vi "HipExo.vi"() -> ()   [LabVIEW 2021]
uses:
  <vilib>/myRIO/Instrument Drivers/Onboard IO/I2C/typedefs/I2C User Configuration.ctl
  <vilib>/myRIO/Instrument Drivers/Onboard IO/I2C/typedefs/I2C Transfer Rate.ctl
  state_typedef.ctl
  <vilib>/Platform/TimedLoop/XDataNode/timing_clust.ctl
  <vilib>/Platform/TimedLoop/XDataNode/nitl_modes.ctl
  <vilib>/Platform/TimedLoop/XDataNode/wakeup.ctl
  <vilib>/myRIO/Instrument Drivers/Onboard IO/PWM/typedefs/PWM Reference.ctl
  <vilib>/myRIO/Common/Instrument Driver Framework/Utilities/typedefs/myRIO Generic Hardware Reference.ctl
  <vilib>/myRIO/Common/Instrument Driver Framework/Utilities/typedefs/Hardware Version Enum.ctl
  <vilib>/myRIO/Common/Instrument Driver Framework/Utilities/typedefs/myRIO v1.0 Reference.ctl
  <vilib>/myRIO/Common/Instrument Driver Framework/Utilities/typedefs/Generic FPGA Reference.ctl
  <vilib>/myRIO/Common/Instrument Driver Framework/myRIO v1.0/PWM/typedefs/PWM Channels Enum.ctl
  <vilib>/myRIO/Instrument Drivers/Onboard IO/PWM/typedefs/PWM Configuration.ctl
  <vilib>/userDefined/High Color/nirio_resource_hc.ctl
  <vilib>/myRIO/Common/Instrument Driver Framework/Utilities/vis/Is FPGA Ref Available.vi
  <vilib>/myRIO/Common/Instrument Driver Framework/myRIO v1.0/PWM/vis/myRIO v1.1 Open PWM.vi
  <vilib>/myRIO/Instrument Drivers/Onboard IO/PWM/vis/Set Duty Cycle and Frequency.vi
  <vilib>/myRIO/Common/Instrument Driver Framework/myRIO v1.0/DIO/vis/myRIO v1.1 Open DIO.vi
  <vilib>/myRIO/Common/Instrument Driver Framework/myRIO v1.0/I2C/vis/myRIO v1.1 Open I2C.vi
  <vilib>/myRIO/Common/Instrument Driver Framework/Utilities/vis/Validate Channels.vi
  <vilib>/myRIO/Common/Instrument Driver Framework/myRIO v1.0/PWM/vis/myRIO v1.0 Reserve PWM.vi
  <vilib>/myRIO/Common/Instrument Driver Framework/myRIO v1.0/UART/vis/myRIO v1.0 Close UART.vi
  <vilib>/myRIO/Common/Instrument Driver Framework/myRIO v1.0/DIO/vis/myRIO v1.0 Reserve DIO.vi
  <vilib>/myRIO/Common/Instrument Driver Framework/myRIO v1.0/I2C/vis/myRIO v1.0 Reserve I2C.vi
  <vilib>/myRIO/Common/Instrument Driver Framework/myRIO v1.0/PWM/vis/myRIO v1.0 Build MUX Configuration PWM.vi
  <vilib>/myRIO/Common/Instrument Driver Framework/myRIO v1.0/Resource Manager/vis/myRIO v1.0 Reserve Channel List.vi
  <vilib>/myRIO/Common/Instrument Driver Framework/myRIO v1.0/DIO/vis/myRIO v1.0 Build MUX Configuration DIO.vi
  <vilib>/myRIO/Common/Instrument Driver Framework/myRIO v1.0/I2C/vis/myRIO v1.0 Build MUX Configuration I2C.vi
  <vilib>/myRIO/Common/Instrument Driver Framework/myRIO v1.0/Resource Manager/vis/myRIO v1.0 Create Configuration List.vi
  <vilib>/myRIO/Common/Instrument Driver Framework/myRIO v1.0/Resource Manager/vis/myRIO v1.0 Reserve Channel.vi
  <vilib>/myRIO/Common/Instrument Driver Framework/myRIO v1.0/Resource Manager/vis/myRIO v1.0 Unreserve Channel.vi
  <vilib>/myRIO/Common/Instrument Driver Framework/myRIO v1.0/Resource Manager/vis/myRIO v1.0 Build Mutex Name.vi
  <vilib>/Utility/VariantDataType/GetNumericInfo.vi
  <vilib>/Utility/error.llb/Error Cluster From Error Code.vi
  <vilib>/myRIO/Common/Instrument Driver Framework/myRIO v1.0/myRIO v1.1 Open.vi
  <vilib>/myRIO/Common/Instrument Driver Framework/Utilities/vis/IO Manager.vi
  <vilib>/myRIO/Common/Instrument Driver Framework/Utilities/vis/Configuration Manager.vi
  <vilib>/myRIO/Common/Instrument Driver Framework/myRIO v1.0/Resource Manager/vis/myRIO v1.0 Configure IO.vi
  <vilib>/myRIO/Common/Instrument Driver Framework/myRIO v1.0/myRIO v1.0 Close.vi
  <vilib>/myRIO/Common/Instrument Driver Framework/myRIO v1.0/I2C/vis/myRIO v1.0 Configure I2C.vi
  <vilib>/myRIO/Common/Instrument Driver Framework/myRIO v1.0/I2C/vis/myRIO v1.0 Write I2C.vi
  <vilib>/myRIO/Common/Instrument Driver Framework/myRIO v1.0/DIO/vis/myRIO v1.0 Write DIO.vi
  <vilib>/myRIO/Common/Instrument Driver Framework/myRIO v1.0/PWM/vis/myRIO v1.0 Write PWM.vi
  <vilib>/myRIO/Common/Instrument Driver Framework/Utilities/vis/FPGA Ref Manager.vi
  <vilib>/myRIO/Common/Instrument Driver Framework/myRIO v1.0/myRIO v1.0 Reset FPGA.vi
  <vilib>/myRIO/Common/Instrument Driver Framework/myRIO v1.0/IRQ/vis/myRIO v1.0 IRQ Info FGV.vi
  <vilib>/myRIO/Common/Instrument Driver Framework/myRIO v1.0/IRQ/vis/myRIO v1.0 Timer IRQ Info FGV.vi
  <vilib>/myRIO/Common/Instrument Driver Framework/myRIO v1.0/IRQ/vis/myRIO v1.0 ISR Agent.vi
  <vilib>/myRIO/Instrument Drivers/Utilities/vis/Reset Index.vi
  <vilib>/myRIO/Common/Instrument Driver Framework/myRIO v1.0/Resource Manager/vis/myRIO v1.0 Block Write Resource Manager.vi
  <vilib>/Platform/TimedLoop/XDataNode/XDataNode.xnode
  <vilib>/myRIO/Express VI/Onboard IO/PWM/PWM Express VI.xnode
  <vilib>/myRIO/Instrument Drivers/Onboard IO/PWM/vis/myRIO PWM Open.xnode
  <vilib>/myRIO/Instrument Drivers/Onboard IO/I2C/I2C.lvlib
  <vilib>/myRIO/Instrument Drivers/Utilities/Utilities.lvlib
  <vilib>/myRIO/Instrument Drivers/Onboard IO/DIO/DIO.lvlib
  <vilib>/Platform/TimedLoop/XDataNode/XDNodeRunTimeDep.lvlib
  <vilib>/myRIO/Instrument Drivers/Onboard IO/PWM/PWM.lvlib
panel:
  out "Numeric":dbl
  in  "error in (no error)":errorcluster
  in  "reset integrator 2":bool
  out "Z displacement 2":dbl format="%#_5g"
  out "Y displacement 2":dbl format="%#_5g"
  out "X displacement 2":dbl format="%#_5g"
  out "Angular displacement [LSB] 2":cluster{dbl, dbl, dbl, dbl}(graph)
  out "Angular rate [LSB/sec] 2":T1(graph)
  out "Z rate 2":dbl format="%.2f"
  out "Y rate 2":dbl format="%.2f"
  out "X rate 2":dbl format="%.2f"
  in  "[ESC]":bool
  out "X":i16
  out "Y":i16
  out "Z":i16
  out "Accelerometer Readings":cluster{i16, i16, i16}(graph)
  out "INT_SOURCE":bool[](array[boolean])
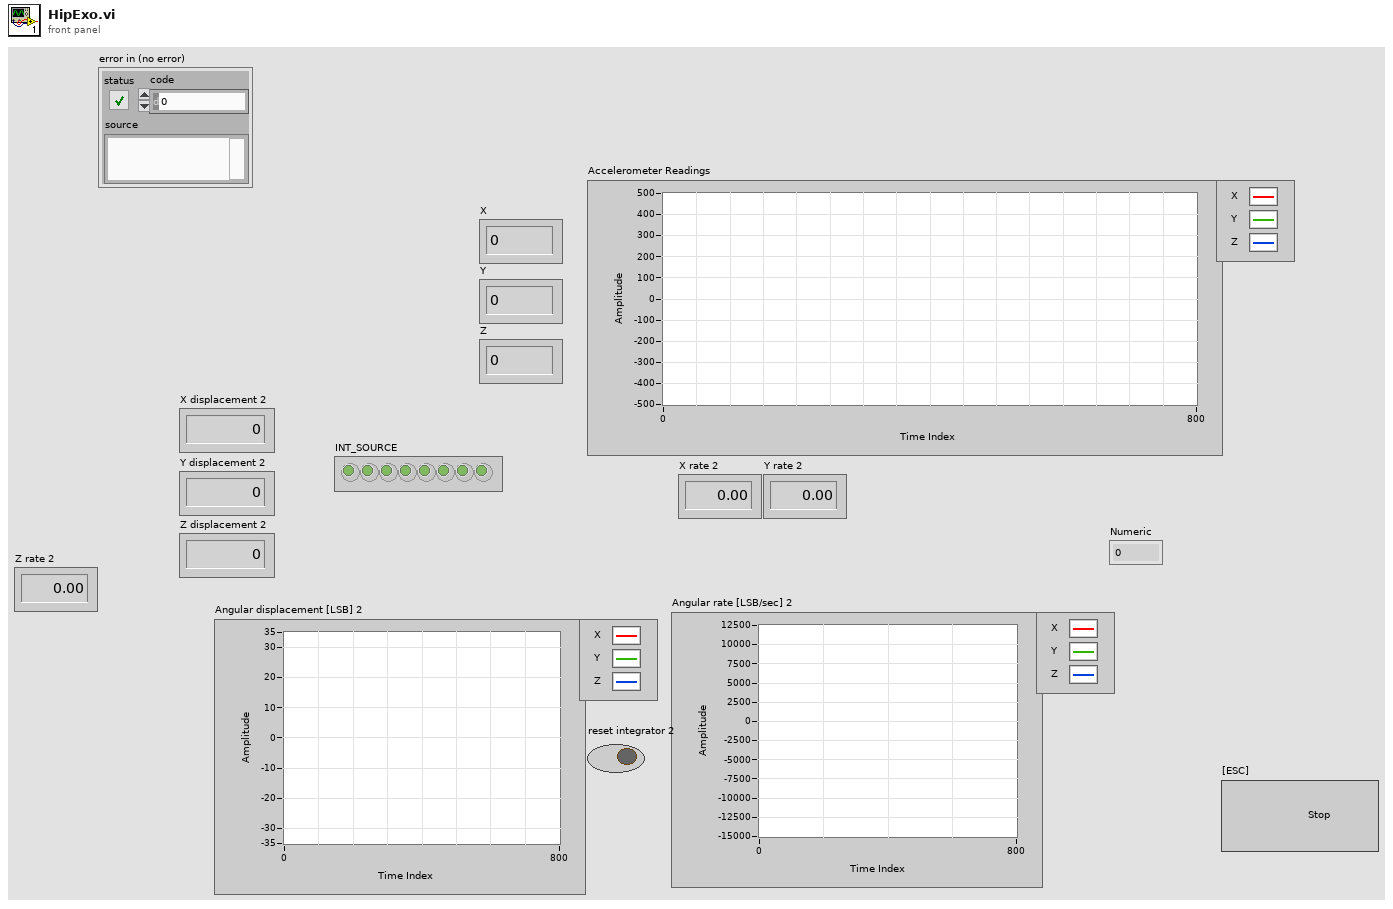
[diagram p1: front panel]
types:
  T1 = cluster{"Numeric 3":dbl, "Numeric 2":dbl, "Numeric":dbl}
  T2 = typedef "state_typedef.ctl" = enum16{"Stair Down", "Stair Up", "Level Walking"}
  T3 = typedef "I2C.lvlib/I2C User Configuration.ctl" = cluster{"I2C Transfer Rate":T4}
  T4 = typedef "I2C.lvlib/I2C Transfer Rate.ctl" = enum16{"Standard mode (100 kbps)", "Fast mode (400 kbps)"}
  T5 = typedef "I2C.lvlib/I2C Reference.ctl" = cluster{"myRIO Reference":T6, "I2C Channels Enum":T10, "I2C Configuration":T11}
  T6 = typedef "myRIO Generic Hardware Reference.ctl" = cluster{"myRIO Model":T7, "myRIO Hardware Reference":T8}
  T7 = typedef "Hardware Version Enum.ctl" = enum16{"Unknown", "myRIO-1900", "myRIO-1950", "roboRIO", "NI ELVIS RIO CM", "ELVIS III"}
  T8 = typedef "myRIO v1.0 Reference.ctl" = cluster{"Generic FPGA Reference":T9, "Allow multiple opens":bool}
  T9 = typedef "Generic FPGA Reference.ctl" = refnum<k20>
  T10 = typedef "I2C Channels Enum.ctl" = enum16{"Not Connected", "A/I2C", "B/I2C", "I2C/I2C"}
  T11 = typedef "I2C.lvlib/I2C Configuration.ctl" = cluster{"I2C Transfer Rate":T4}
  T12 = typedef "DIO.lvlib/DIO Reference.ctl" = cluster{"myRIO Reference":T6, "DIO Channels List":T13}
  T13 = typedef "DIO Channels List.ctl" = T14[]
  T14 = typedef "DIO Channels Enum.ctl" = enum16{"Not Connected", "C/DIO0", "C/DIO1", "C/DIO2", "C/DIO3", "C/DIO4", "C/DIO5", "C/DIO6", "C/DIO7", "A/DIO0", "A/DIO1", "A/DIO2", "A/DIO3", "A/DIO4", "A/DIO5", "A/DIO6", "A/DIO7", "A/DIO8", "A/DIO9", "A/DIO10", "A/DIO11", "A/DIO12", "A/DIO13", "A/DIO14", "A/DIO15", "A/DIO16", "A/DIO17", "A/DIO18", "A/DIO19", "B/DIO0", "B/DIO1", "B/DIO2", "B/DIO3", "B/DIO4", "B/DIO5", "B/DIO6", "B/DIO7", "B/DIO8", "B/DIO9", "B/DIO10", "B/DIO11", "B/DIO12", "B/DIO13", "B/DIO14", "B/DIO15", "B/DIO16", "B/DIO17", "B/DIO18", "B/DIO19", "LED0", "LED1", "LED2", "LED3", "Button0", "DIO/DIO0", "DIO/DIO1", "DIO/DIO2", "DIO/DIO3", "DIO/DIO4", "DIO/DIO5", "DIO/DIO6", "DIO/DIO7", "DIO/DIO8", "DIO/DIO9", "SPI/CS0", "SPI/CS1", "SPI/CS2", "SPI/CS3", "LED RADIO (Green)", "LED RADIO (Red)", "LED COMM (Green)", "LED COMM (Red)", "LED MODE (Green)", "LED MODE (Red)"}
  T15 = typedef "XDNodeRunTimeDep.lvlib/timing_clust.ctl" = cluster{"Expected End [f-1]":u64, "Actual End [f-1]":u64, "Finished Late? [f-1]":bool, "Expected End [i-1]":u64, "Actual End [i-1]":u64, "Finished Late? [i-1]":bool, "Expected Start [i]":u64, "Actual Start [i]":u64, "Expected Start [f]":u64, "Actual Start [f]":u64, "Source Name":string, "Structure Name":string, "Period":i64, "Deadline":i64, "Offset":i64, "Start":i64, "Priority":i32, "Timeout":i32, "Mode":T16, "Wakeup Reason":T17, "Error":errorcluster, "Source Type":string, "Secondary Source Type":string, "Global End Time":u64, "Global Start Time":u64, "Frame Duration":u64, "Iteration Duration":u64, "Assigned CPU":i32, "I/O Scan Engine Mode":u32}
  T16 = typedef "XDNodeRunTimeDep.lvlib/nitl_modes.ctl" = enum32{"No Change", "Process missed periods, maintain original phase", "Discard missed periods, maintain original phase", "Process missed periods, ignore original phase", "Discard missed periods, ignore original phase"}
  T17 = typedef "XDNodeRunTimeDep.lvlib/wakeup.ctl" = enum32{"Normal", "Aborted", "Asynchronous wakeup", "Timing source error", "Timed loop error", "Timeout"}
  T18 = typedef "PWM.lvlib/PWM Reference.ctl" = cluster{"myRIO Reference":T6, "PWM Channels Enum":T19, "PWM Configuration":T20}
  T19 = typedef "PWM Channels Enum.ctl" = enum16{"Not Connected", "C/PWM0", "C/PWM1", "A/PWM0", "A/PWM1", "A/PWM2", "A/PWM3", "A/PWM4", "A/PWM5", "A/PWM6", "A/PWM7", "A/PWM8", "A/PWM9", "A/PWM10", "A/PWM11", "A/PWM12", "A/PWM13", "A/PWM14", "A/PWM15", "A/PWM16", "A/PWM17", "A/PWM18", "A/PWM19", "B/PWM0", "B/PWM1", "B/PWM2", "B/PWM3", "B/PWM4", "B/PWM5", "B/PWM6", "B/PWM7", "B/PWM8", "B/PWM9", "B/PWM10", "B/PWM11", "B/PWM12", "B/PWM13", "B/PWM14", "B/PWM15", "B/PWM16", "B/PWM17", "B/PWM18", "B/PWM19", "PWM/PWM0", "PWM/PWM1", "PWM/PWM2", "PWM/PWM3", "PWM/PWM4", "PWM/PWM5", "PWM/PWM6", "PWM/PWM7", "PWM/PWM8", "PWM/PWM9"}
  T20 = typedef "PWM.lvlib/PWM Configuration.ctl" = cluster{"Frequency":dbl, "Duty Cycle":dbl}
  T21 = typedef "nirio_resource_hc.ctl" = tag
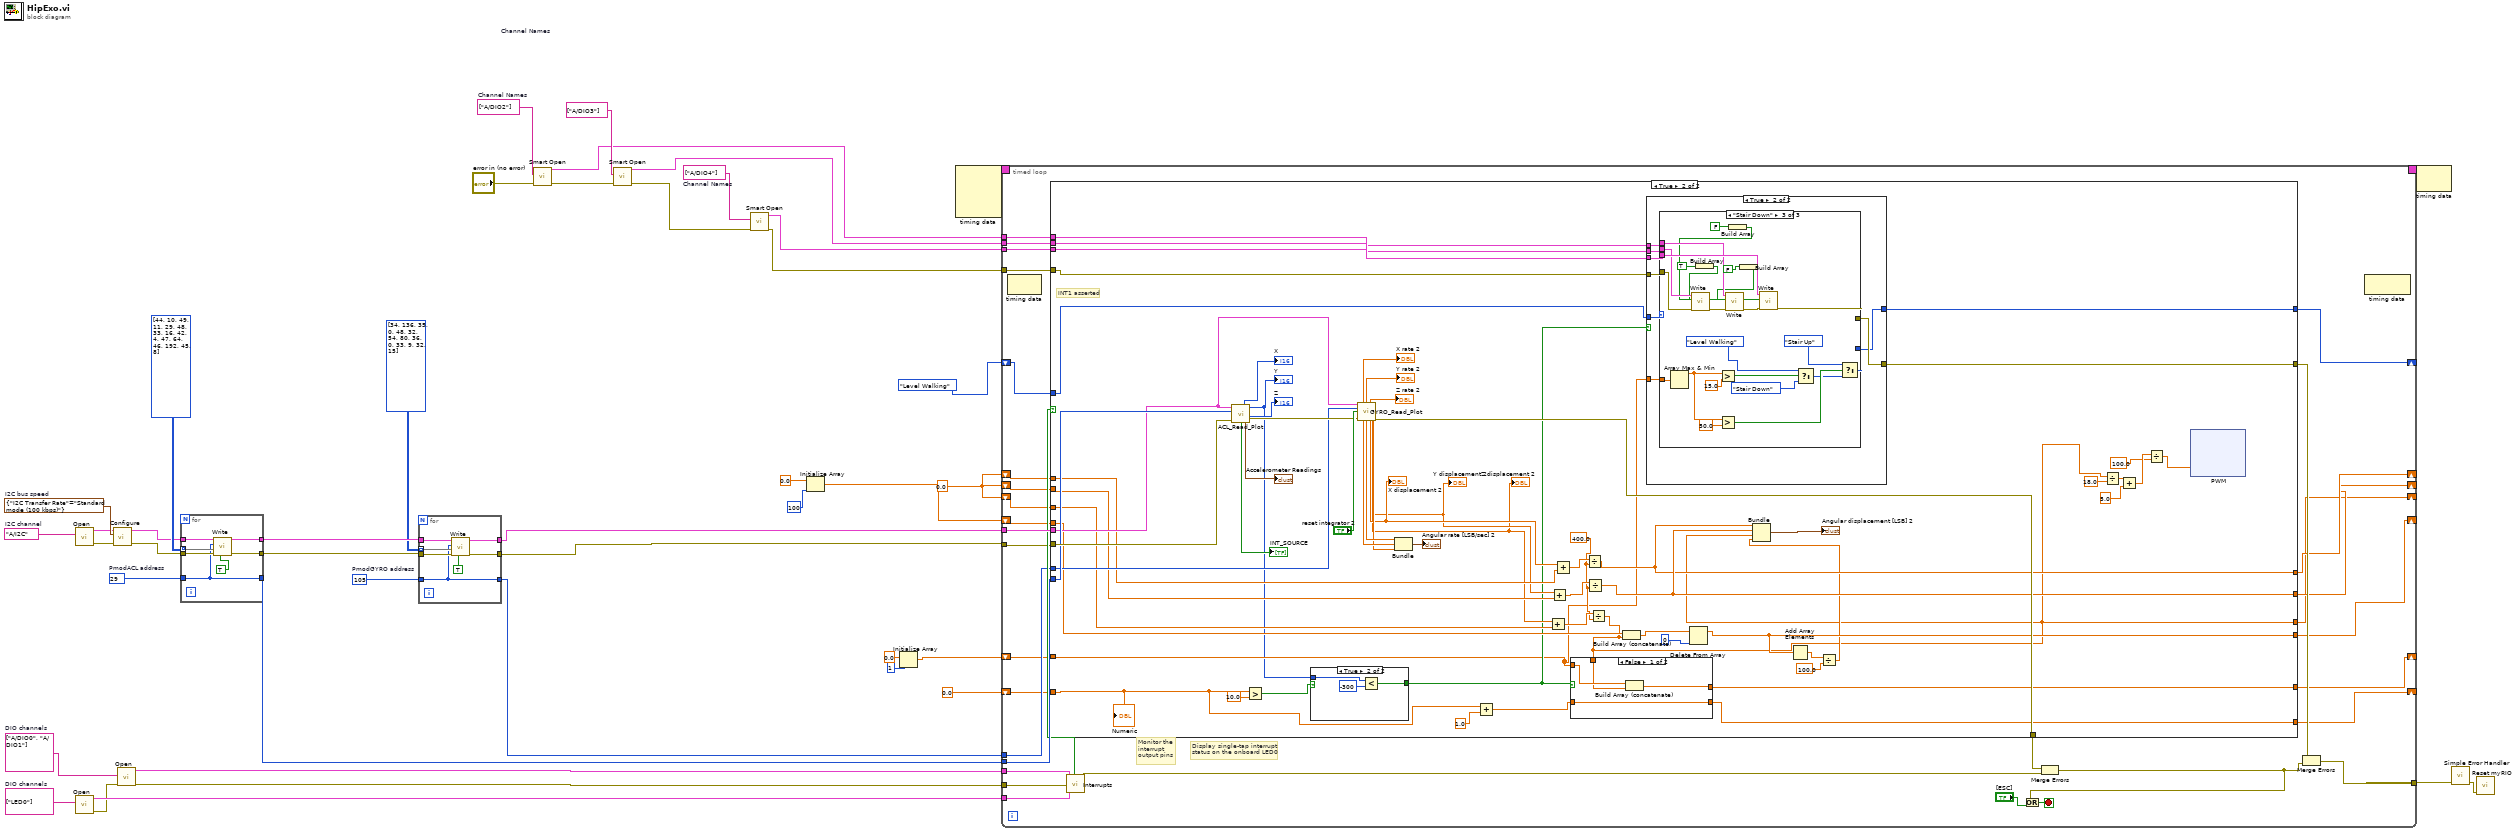
[diagram p0: block diagram]
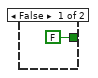
[diagram p3: hidden frame]
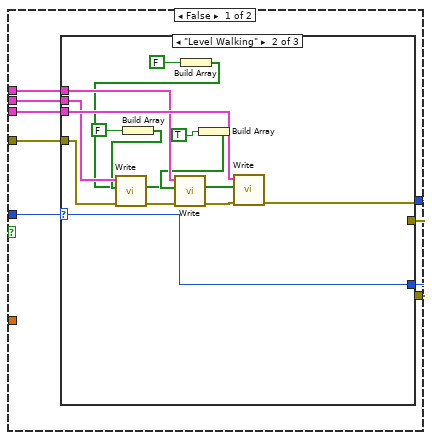
[diagram p4: hidden frame]
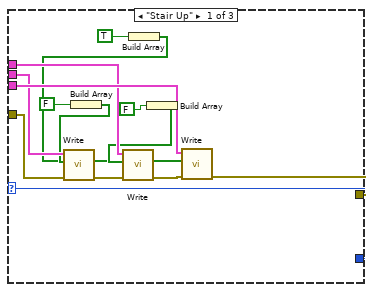
[diagram p5: hidden frame]
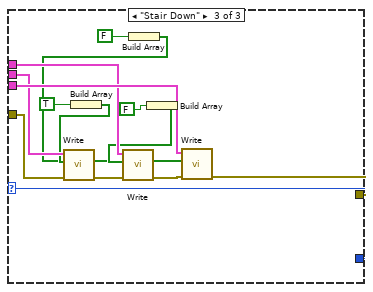
[diagram p6: hidden frame]
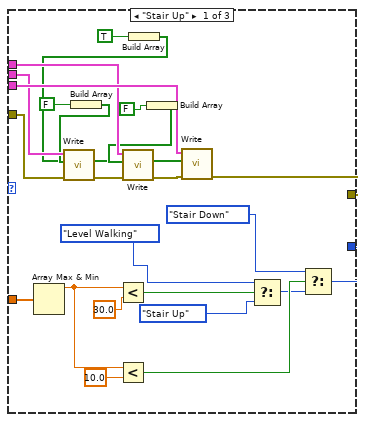
[diagram p7: hidden frame]
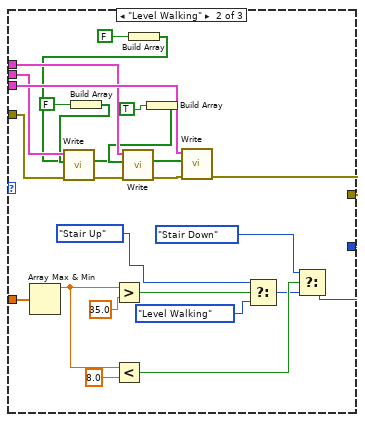
[diagram p8: hidden frame]
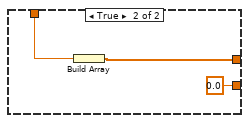
[diagram p9: hidden frame]
diagram:
  w9 = 0.0
  w16 = tag[] ["A/DIO3"]  # Channel Names
  w17 = tag[] ["A/DIO4"]  # Channel Names
  w19 = tag[] ["A/DIO2"]  # Channel Names
  w23 = u8 105  # PmodGYRO address
  w29 = tag[] ["LED0"]  # DIO channels
  w30 = tag[] ["A/DIO0", "A/DIO1"]  # DIO channels
  w40 = T3 {"I2C Transfer Rate"=enum."Standard mode (100 kbps)"}  # I2C bus speed
  w41 = tag "A/I2C"  # I2C channel
  w33 = u8 29  # PmodACL address
  n1 = call <vilib>:"Open.vi"("Channel Name"=w41) -> ("error out"=w38:errorcluster, "I2C Ref Out"=w39:T5)  [unwired: 9 in]
  n2 = call <vilib>:"Open.vi"("Channel Names"=w29) -> ("error out"=w27:errorcluster, "DIO Ref Out"=w28:T12)  [unwired: 9 in]
  n3 = call <vilib>:"Configure.vi"("error in (no error)"=w38, "I2C User Configuration"=w40, "I2C Ref In"=w39) -> ("error out"=w34:errorcluster, "I2C Ref Out"=w35:T5)  [unwired: 7 in]
  n4 = call <vilib>:"Open.vi"("error in (no error)"=w27, "Channel Names"=w30) -> ("error out"=w32:errorcluster, "DIO Ref Out"=w31:T12)  [unwired: 8 in]
  n5 = for {
    tunnel: [w52] -> w25
    tunnel: [w51] -> w26
    tunnel: [w47] -> w37
    tunnel: u8[][] [[44, 10], [49, 11], [29, 48], [33, 16], [42, 4], [47, 64], [46, 192], [45, 8]] ("Bytes to Write") -> [w50] mode=indexing
    tunnel: w35 -> [w49]
    tunnel: w34 -> [w48]
    tunnel: w33 -> [w47]
    n6 = call <vilib>:"Write.vi"("Keep Bus Busy"=TRUE, "error in (no error)"=w48, "Bytes to Write"=w50, "Slave Address (7-bit)"=w47, "I2C Ref In"=w49) -> ("error out"=w52:errorcluster, "I2C Ref Out"=w51:T5)  [unwired: 5 in]
  }
  n7 = for {
    tunnel: [w59] -> w21
    tunnel: [w58] -> w20
    tunnel: [w54] -> w22
    tunnel: u8[][] [[34, 136], [35, 0], [48, 32], [54, 80], [36, 0], [33, 9], [32, 15]] ("Bytes to Write") -> [w57] mode=indexing
    tunnel: w26 -> [w56]
    tunnel: w25 -> [w55]
    tunnel: w23 -> [w54]
    n8 = call <vilib>:"Write.vi"("Keep Bus Busy"=TRUE, "error in (no error)"=w55, "Bytes to Write"=w57, "Slave Address (7-bit)"=w54, "I2C Ref In"=w56) -> ("error out"=w59:errorcluster, "I2C Ref Out"=w58:T5)  [unwired: 5 in]
  }
  n9 = call <vilib>:"Smart Open.vi"("error in (no error)"="error in (no error)", "Channel Names"=w19) -> ("error out"=w15:errorcluster, "DIO Ref Out"=w10:T12)  [unwired: 8 in]
  n10 = call <vilib>:"Smart Open.vi"("error in (no error)"=w15, "Channel Names"=w16) -> ("error out"=w14:errorcluster, "DIO Ref Out"=w11:T12)  [unwired: 8 in]
  n11 = call <vilib>:"Smart Open.vi"("error in (no error)"=w14, "Channel Names"=w17) -> ("error out"=w13:errorcluster, "DIO Ref Out"=w12:T12)  [unwired: 8 in]
  n12 = Initialize Array(0.0, 100) -> (w6:dbl[])
  n13 = Initialize Array(0.0 ("element"), 1 ("dimension size")) -> (w2:dbl[])
  n14 = node-c288() -> (w45:T15)  [unwired: 4 in]
  n15 = timed-loop {
    tunnel: [w78] -> w42
    tunnel: w37 -> [w89]
    tunnel: w32 -> [w88]
    tunnel: w31 -> [w87]
    timing: w45 -> [_]
    timing-out: [_] -> w44
    tunnel: w28 -> [w84]
    tunnel: w21 -> [w82]
    tunnel: w22 -> [w81]
    shift-right: [w80] -> _
    shift-left: state_typedef."Level Walking" -> [w72]
    tunnel: w13 -> [w79]
    tunnel: w12 -> [w75]
    tunnel: w11 -> [w74]
    tunnel: w10 -> [w73]
    tunnel: w20 -> [w90]
    shift-right: [w70] -> _
    shift-left: w9 -> [w71]
    shift-right: [w67] -> _
    shift-left: w9 -> [w69]
    shift-right: [w66] -> _
    shift-left: w9 -> [w68]
    shift-right: [w64] -> _
    shift-left: w6 -> [w65]
    shift-right: [w62] -> _
    shift-left: w2 -> [w63]
    shift-right: [w60] -> _
    shift-left: 0.0 -> [w61]
    stop <- w92 stop-if-true
    # "Display single-tap interrupt\nstatus on the onboard LED0"
    # "Monitor the\ninterrupt\noutput pins"
    n16 = node-c288() -> ()  [unwired: 1 in, 1 out]
    n17 = call "Interrupts.vi"("error in (no error)"=w88, "DIO Ref Out"=w84, "DIO Ref Out 2"=w87) -> ("error out"=w83:errorcluster, "INT1"=w85:bool)  [unwired: 7 in]
    n18 = case shown="True" w85 {
      tunnel: w82 -> [w103 w164]
      tunnel: w90 -> [_ w150]
      tunnel: w89 -> [_ w163]
      tunnel: [w103 w149] -> w86
      tunnel: w81 -> [_ w151]
      tunnel: w72 -> [w102 w148]
      tunnel: [w102 w147] -> w80
      tunnel: w79 -> [w101 w146]
      tunnel: [w101 w145] -> w76
      tunnel: w75 -> [_ w144]
      tunnel: w74 -> [_ w143]
      tunnel: w73 -> [_ w142]
      tunnel: w71 -> [w100 w141]
      tunnel: [w100 w131] -> w70
      tunnel: w69 -> [w99 w139]
      tunnel: w68 -> [w98 w138]
      tunnel: [w99 w133] -> w67
      tunnel: [w98 w111] -> w66
      tunnel: w65 -> [w97 w129]
      tunnel: [w97 w126] -> w64
      tunnel: w63 -> [w96 w121]
      tunnel: [w96 w114] -> w62
      tunnel: w61 -> [w95 w108]
      tunnel: [w95 w110] -> w60
      frame False {
        # "INT1 deasserted"
      }
      frame True {
        w130 = 400.0
        # "INT1 asserted"
        n19 = call "ACL_Read_Plot.vi"("error in (no error)"=w164, "PmodACL address"=w163, "I2C Ref Out"=w150) -> ("error out"=w152:errorcluster, "Numeric 3"=→"Z":i16, "Array"=→"INT_SOURCE":bool[], "Numeric"=w104:i16, "Cluster"=→"Accelerometer Readings":cluster{i16, i16, i16}, "Numeric 2"=→"X":i16)  [unwired: 3 in]
        "Y" <- w104
        n20 = Greater?(x=w108, y=10.0) -> (0:w113:bool)
        n21 = case shown="True" w113 {
          tunnel: [FALSE w168] -> w122
          tunnel: w104 -> [_ w167]
          frame False {
          }
          frame True {
            n22 = Less?(x=w167, y=i16 -300) -> (x < y?=w168:bool)
          }
        }
        n23 = call "GYRO_Read_Plot.vi"("I2C Ref Out"=w150, "PmodGYRO address"=w151, "reset integrator"="reset integrator 2", "error in (no error)"=w152) -> ("X rate"=→"X rate 2":dbl, "Y rate"=→"Y rate 2":dbl, "integral x(t)"=w140:dbl, "integral x(t) 3"=w137:dbl, "Numeric"=w157:dbl, "integral x(t) 2"=w136:dbl, "Numeric 2"=w158:dbl, "Numeric 3"=w160:dbl, "Z rate"=→"Z rate 2":dbl, "error out"=w149:errorcluster)  [unwired: 1 in, 1 out]
        "X displacement 2" <- w140
        "Y displacement 2" <- w137
        "Z displacement 2" <- w136
        n24 = Bundle "Bundle"("Numeric 3"=w160, "Numeric 2"=w158, "Numeric"=w157) -> (→"Angular rate [LSB/sec] 2":T1)  [unwired: 1 in]
        n25 = Add(x=w108, y=1.0) -> (x+y=w107:dbl)
        n26 = Add(x=w136, y=w138) -> (x+y=w135:dbl)
        n27 = Add(x=w137, y=w139) -> (x+y=w134:dbl)
        n28 = Add(x=w140, y=w141) -> (x+y=w132:dbl)
        n29 = Divide(x=w132, y=w130) -> (x/y=w131:dbl)
        n30 = Divide(x=w134, y=w130) -> (x/y=w133:dbl)
        n31 = Divide(x=w135, y=w130) -> (x/y=w111:dbl)
        n32 = case shown="False" w122 {
          tunnel: w121 -> [w337 _]
          tunnel: w111 -> [w336 w340]
          tunnel: [w335 w339] -> w114
          tunnel: w107 -> [w334 _]
          tunnel: [w334 0.0] -> w110
          frame False {
            n33 = Build Array (concatenate)(w337, w336) -> (w335:dbl[])
          }
          frame True {
            n34 = Build Array(w340) -> (w339:dbl[])
          }
        }
        n35 = Build Array (concatenate)(w129, w111) -> (w128:dbl[])
        n36 = case shown="True" w122 {
          tunnel: w148 -> [w211 w257]
          tunnel: [w210 w255] -> w147
          tunnel: w146 -> [w209 w258]
          tunnel: [w208 w256] -> w145
          tunnel: w144 -> [w207 w259]
          tunnel: w143 -> [w206 w260]
          tunnel: w142 -> [w205 w261]
          tunnel: w121 -> [_ w254]
          frame False {
            n37 = case shown="\"Level Walking\"" w211 {
              selector: w211 -> [w225 w226 w253]
              tunnel: [w225 w226 w253] -> w210
              tunnel: w209 -> [w221 w236 w249]
              tunnel: [w224 w239 w252] -> w208
              tunnel: w207 -> [w223 w238 w251]
              tunnel: w206 -> [w222 w237 w250]
              tunnel: w205 -> [w218 w233 w246]
              frame "Stair Up" {
                n38 = Build Array(FALSE) -> (w216:bool[])
                n39 = call <vilib>:"Write.vi"("error in (no error)"=w221, "Values"=w216, "DIO Ref In"=w222) -> ("error out"=w220:errorcluster)  [unwired: 6 in, 1 out]
                n40 = Build Array(TRUE) -> (w212:bool[])
                n41 = Build Array(FALSE) -> (w214:bool[])
                n42 = call <vilib>:"Write.vi"("error in (no error)"=w220, "Values"=w214, "DIO Ref In"=w218) -> ("error out"=w219:errorcluster)  [unwired: 6 in, 1 out]
                n43 = call <vilib>:"Write.vi"("error in (no error)"=w219, "Values"=w212, "DIO Ref In"=w223) -> ("error out"=w224:errorcluster)  [unwired: 6 in, 1 out]
              }
              frame "Level Walking" {
                n44 = Build Array(FALSE) -> (w231:bool[])
                n45 = call <vilib>:"Write.vi"("error in (no error)"=w236, "Values"=w231, "DIO Ref In"=w237) -> ("error out"=w235:errorcluster)  [unwired: 6 in, 1 out]
                n46 = Build Array(FALSE) -> (w227:bool[])
                n47 = Build Array(TRUE) -> (w229:bool[])
                n48 = call <vilib>:"Write.vi"("error in (no error)"=w235, "Values"=w229, "DIO Ref In"=w233) -> ("error out"=w234:errorcluster)  [unwired: 6 in, 1 out]
                n49 = call <vilib>:"Write.vi"("error in (no error)"=w234, "Values"=w227, "DIO Ref In"=w238) -> ("error out"=w239:errorcluster)  [unwired: 6 in, 1 out]
              }
              frame "Stair Down" {
                n50 = Build Array(TRUE) -> (w244:bool[])
                n51 = call <vilib>:"Write.vi"("error in (no error)"=w249, "Values"=w244, "DIO Ref In"=w250) -> ("error out"=w248:errorcluster)  [unwired: 6 in, 1 out]
                n52 = Build Array(FALSE) -> (w240:bool[])
                n53 = Build Array(FALSE) -> (w242:bool[])
                n54 = call <vilib>:"Write.vi"("error in (no error)"=w248, "Values"=w242, "DIO Ref In"=w246) -> ("error out"=w247:errorcluster)  [unwired: 6 in, 1 out]
                n55 = call <vilib>:"Write.vi"("error in (no error)"=w247, "Values"=w240, "DIO Ref In"=w251) -> ("error out"=w252:errorcluster)  [unwired: 6 in, 1 out]
              }
            }
          }
          frame True {
            n56 = case shown="\"Stair Down\"" w257 {
              tunnel: [w262 w286 w310] -> w255
              tunnel: w258 -> [w282 w306 w330]
              tunnel: [w285 w309 w333] -> w256
              tunnel: w259 -> [w284 w308 w332]
              tunnel: w260 -> [w283 w307 w331]
              tunnel: w261 -> [w279 w303 w327]
              tunnel: w254 -> [w263 w292 w311]
              frame "Stair Up" {
                n57 = Array Max & Min(array=w263) -> (max value=w268:dbl)  [unwired: 3 out]
                n58 = Build Array(FALSE) -> (w277:bool[])
                n59 = call <vilib>:"Write.vi"("error in (no error)"=w282, "Values"=w277, "DIO Ref In"=w283) -> ("error out"=w281:errorcluster)  [unwired: 6 in, 1 out]
                n60 = Less?(x=w268, y=30.0) -> (x < y?=w271:bool)
                n61 = Less?(x=w268, y=10.0) -> (x < y?=w266:bool)
                n62 = Build Array(TRUE) -> (w273:bool[])
                n63 = Build Array(FALSE) -> (w275:bool[])
                n64 = call <vilib>:"Write.vi"("error in (no error)"=w281, "Values"=w275, "DIO Ref In"=w279) -> ("error out"=w280:errorcluster)  [unwired: 6 in, 1 out]
                n65 = call <vilib>:"Write.vi"("error in (no error)"=w280, "Values"=w273, "DIO Ref In"=w284) -> ("error out"=w285:errorcluster)  [unwired: 6 in, 1 out]
                n66 = Select(t=state_typedef."Level Walking", s=w271, f=state_typedef."Stair Up") -> (s? t:f=w264:T2)
                n67 = Select(t=state_typedef."Stair Down", s=w266, f=w264) -> (s? t:f=w262:T2)
              }
              frame "Level Walking" {
                n68 = Array Max & Min(array=w292) -> (max value=w291:dbl)  [unwired: 3 out]
                n69 = Build Array(FALSE) -> (w301:bool[])
                n70 = call <vilib>:"Write.vi"("error in (no error)"=w306, "Values"=w301, "DIO Ref In"=w307) -> ("error out"=w305:errorcluster)  [unwired: 6 in, 1 out]
                n71 = Greater?(x=w291, y=35.0) -> (0:w295:bool)
                n72 = Less?(x=w291, y=8.0) -> (x < y?=w289:bool)
                n73 = Build Array(FALSE) -> (w297:bool[])
                n74 = Build Array(TRUE) -> (w299:bool[])
                n75 = call <vilib>:"Write.vi"("error in (no error)"=w305, "Values"=w299, "DIO Ref In"=w303) -> ("error out"=w304:errorcluster)  [unwired: 6 in, 1 out]
                n76 = call <vilib>:"Write.vi"("error in (no error)"=w304, "Values"=w297, "DIO Ref In"=w308) -> ("error out"=w309:errorcluster)  [unwired: 6 in, 1 out]
                n77 = Select(t=state_typedef."Stair Up", s=w295, f=state_typedef."Level Walking") -> (s? t:f=w287:T2)
                n78 = Select(t=state_typedef."Stair Down", s=w289, f=w287) -> (s? t:f=w286:T2)
              }
              frame "Stair Down" {
                n79 = Array Max & Min(array=w311) -> (max value=w316:dbl)  [unwired: 3 out]
                n80 = Build Array(TRUE) -> (w325:bool[])
                n81 = call <vilib>:"Write.vi"("error in (no error)"=w330, "Values"=w325, "DIO Ref In"=w331) -> ("error out"=w329:errorcluster)  [unwired: 6 in, 1 out]
                n82 = Greater?(x=w316, y=15.0) -> (0:w319:bool)
                n83 = Greater?(x=w316, y=50.0) -> (0:w314:bool)
                n84 = Build Array(FALSE) -> (w321:bool[])
                n85 = Build Array(FALSE) -> (w323:bool[])
                n86 = call <vilib>:"Write.vi"("error in (no error)"=w329, "Values"=w323, "DIO Ref In"=w327) -> ("error out"=w328:errorcluster)  [unwired: 6 in, 1 out]
                n87 = call <vilib>:"Write.vi"("error in (no error)"=w328, "Values"=w321, "DIO Ref In"=w332) -> ("error out"=w333:errorcluster)  [unwired: 6 in, 1 out]
                n88 = Select(t=state_typedef."Level Walking", s=w319, f=state_typedef."Stair Down") -> (s? t:f=w312:T2)
                n89 = Select(t=state_typedef."Stair Up", s=w314, f=w312) -> (s? t:f=w310:T2)
              }
            }
          }
        }
        n90 = Delete From Array(array=w128, index=0) -> (array with subset deleted=w126:dbl[])  [unwired: 1 in, 1 out]
        n91 = Add Array Elements(numeric array=w126) -> (sum=w125:dbl)
        n92 = Divide(x=w125, y=100.0) -> (x/y=w123:dbl)
        n93 = Bundle "Bundle"(w131, w133, w111, w123) -> (→"Angular displacement [LSB] 2":cluster{dbl, dbl, dbl, dbl})  [unwired: 1 in]
        n94 = Divide(x=w111, y=18.0) -> (x/y=w118:dbl)
        n95 = Add(x=w118, y=5.0) -> (x+y=w120:dbl)
        n96 = Divide(x=w120, y=100.0) -> (x/y=w119:dbl)
        n97 = xnode "PWM"("Duty Cycle"=w119) -> ()  [unwired: 1 in, 1 out]
        "Numeric" <- w108
      }
    }
    n98 = Merge Errors "Merge Errors"(w86, w83) -> (w77:errorcluster)
    n99 = Or(x=w77, y="[ESC]") -> (x .or. y?=w92:bool)
    n100 = Merge Errors "Merge Errors"(w76, w77) -> (w78:errorcluster)
    n101 = node-c288() -> ()  [unwired: 1 in, 1 out]
  }
  n102 = node-c288(w44) -> ()  [unwired: 1 out]
  n103 = call <vilib>:"Simple Error Handler.vi"("error in (no error)"=w42) -> ("error out"=w43:errorcluster)  [unwired: 4 in, 4 out]
  n104 = call <vilib>:"Reset myRIO.vi"("error in (no error)"=w43) -> ()  [unwired: 10 in, 1 out]
